vi "Team195_SetVoltageMotorControlOpenCANTalonSRX.vi"(4 "CAN.Max Vout":dbl=12.0, 5 "InverseTransformVIRef":T2, 6 "Invert":bool, 7 "TransformVIRef":T2, 8 "error in (no error)":errorcluster, 9 "Master Device Number":u8, 10 "Device Number":u8, 11 "Control Mode":T1) -> (0 "error out":errorcluster, 3 "MotorControlDeviceRef":T3={"DeviceStatus"={"status"=FALSE, "code"=0, "source"=""}, "Type"=enum."PWM", "PWM"={"Controller"=enum."Controller 1", "PWM Channel"=enum."Invalid", "DeadBand"={"Name"="", "maxPositivePwm"=0, "minPositivePwm"=0, "centerPwm"=0, "maxNegativePwm"=0, "minNegativePwm"=0, "angularRange"=0}}, "CAN"={"Device Number"=0, "Control Mode"=enum."Percent VBus", "Semaphore"=refnum, "Max Vout"=12.0, "TalonSRX Control Mode"=enum."Percent VBus"}, "Invert"=FALSE, "TransformRef"=refnum, "InvTransformRef"=refnum})   [LabVIEW 2014]
doc: "Creates a reference to the Victor motor controller you specify. You must open a reference before using any other VIs on this palette. After you open a reference to the Victor motor controller, you can use the SetOutput and GetOutput VIs to set and get the output voltage of the motor controller, respectively.\n\nThis software is licensed. Open the labview\\readme\\WPI Robotics Library Open Source License.txt file for more information."
uses:
  <vilib>/Rock Robotics/WPI/MotorControl/WPI_MotorControlDeviceRef.ctl
  <vilib>/Rock Robotics/WPI/MotorControl/WPI_MotorControlType.ctl
  <vilib>/Rock Robotics/SystemInterfaces/Typedef/FPGA_TypedefDigitalModule.ctl
  <vilib>/Rock Robotics/SystemInterfaces/DIO/FPGA_DIOPWMChannel.ctl
  <vilib>/Rock Robotics/WPI/PWM/WPI_PWMDeadband.ctl
  <vilib>/Rock Robotics/WPI/CAN/Jaguar/SubVIs/WPI_CANJaguar_ControlMode.ctl
  <vilib>/Rock Robotics/WPI/CAN/TalonSRX/WPI_CANTalonSRX_APIControlMode.ctl
  <vilib>/Rock Robotics/WPI/PWM/WPI_PWMTransform_ConPane.ctl
  <vilib>/Rock Robotics/SystemInterfaces/NetworkCommunication/NetComm_UsageReport_ResourceType.ctl
  <vilib>/Rock Robotics/WPI/CAN/TalonSRX/WPI_CANTalonSRX_GlobalOps.ctl
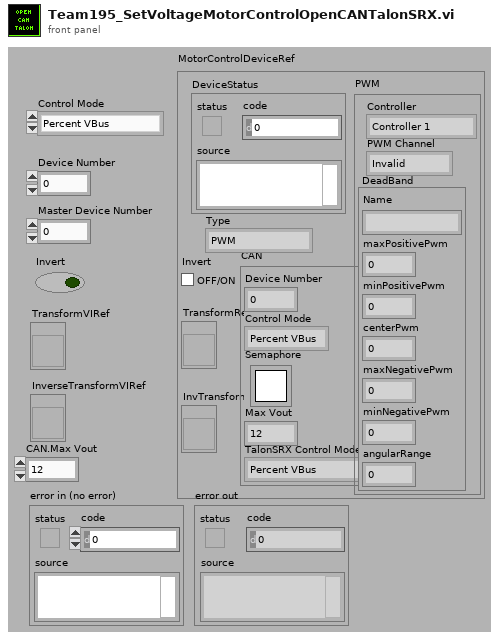
[diagram p1: front panel]
types:
  T1 = typedef "WPI_CANTalonSRX_APIControlMode.ctl" = enum8{"Percent VBus", "Speed", "Position", "Slave", "Unchanged / Invalid"}
  T2 = typedef "WPI_PWMTransform_ConPane.ctl" = refnum<vi>
  T3 = typedef "WPI_MotorControlDeviceRef.ctl" = cluster{"DeviceStatus":errorcluster, "Type":T4, "PWM":cluster{"Controller":T5, "PWM Channel":T6, "DeadBand":T7}, "CAN":cluster{"Device Number":u8, "Control Mode":T8, "Semaphore":T9, "Max Vout":dbl, "TalonSRX Control Mode":T1}, "Invert":bool, "TransformRef":T2, "InvTransformRef":T2}
  T4 = typedef "WPI_MotorControlType.ctl" = enum16{"PWM", "CAN", "CANTalonSRX"}
  T5 = typedef "FPGA_TypedefDigitalModule.ctl" = enum16{"Controller 1"}
  T6 = typedef "FPGA_DIOPWMChannel.ctl" = enum8{"PWM 0", "PWM 1", "PWM 2", "PWM 3", "PWM 4", "PWM 5", "PWM 6", "PWM 7", "PWM 8", "PWM 9", "PWM MXP 0", "PWM MXP 1", "PWM MXP 2", "PWM MXP 3", "PWM MXP 4", "PWM MXP 5", "PWM MXP 6", "PWM MXP 7", "PWM MXP 8", "PWM MXP 9", "Invalid"}
  T7 = typedef "WPI_PWMDeadband.ctl" = cluster{"Name":string, "maxPositivePwm":i32, "minPositivePwm":i32, "centerPwm":i32, "maxNegativePwm":i32, "minNegativePwm":i32, "angularRange":u16}
  T8 = typedef "WPI_CANJaguar_ControlMode.ctl" = enum8{"Percent VBus", "Current", "Speed", "Position", "Voltage"}
  T9 = typedef "Semaphore RefNum" = refnum<k1>
  T10 = typedef "WPI_CANTalonSRX_GlobalOps.ctl" = enum16{"Read For Send", "Write After Receive General", "Write After Receive Feedback", "Write After Receive Encoder", "Write After Receive Ain", "Write Error", "Get All", "Set Output", "Set Mode", "Set Master ID", "Set Brake Mode", "Set Reverse Feedback Sensor", "Set Reverse Closed Loop Output", "Set Override Limits", "Set Forward Limit Enabled", "Set Reverse Limit Enabled", "Set Feedback Select", "Set Profile Select", "Set Throttle Ramp Rate", "Disable"}
  T11 = typedef "NetComm_UsageReport_ResourceType.ctl" = enum8{"Controller", "Module", "Language", "CANPlugin", "Accelerometer", "ADXL345", "AnalogChannel", "AnalogTrigger", "AnalogTriggerOutput", "CANJaguar", "Compressor", "Counter", "Dashboard", "DigitalInput", "DigitalOutput", "DriverStationCIO", "DriverStationEIO", "DriverStationLCD", "Encoder", "GearTooth", "Gyro", "I2C", "Framework", "Jaguar", "Joystick", "Kinect", "KinectStick", "PIDController", "Preferences", "PWM", "Relay", "RobotDrive", "SerialPort", "Servo", "Solenoid", "SPI", "Task", "Ultrasonic", "Victor", "Button", "Command", "AxisCamera", "PCVideoServer", "SmartDashboard", "Talon", "HiTechnicColorSensor", "HiTechnicAccel", "HiTechnicCompass", "SRF08", "AnalogOutput", "Victor SP", "Talon SRX", "CAN Talon SRX"}
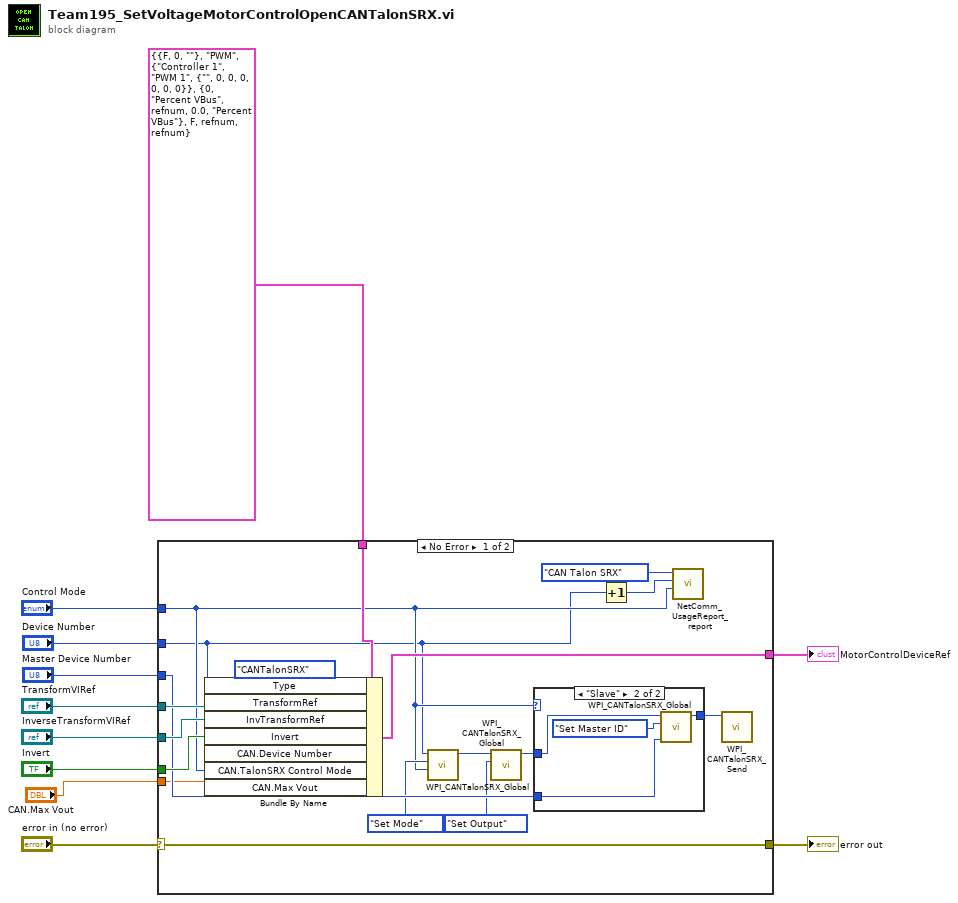
[diagram p0: block diagram]
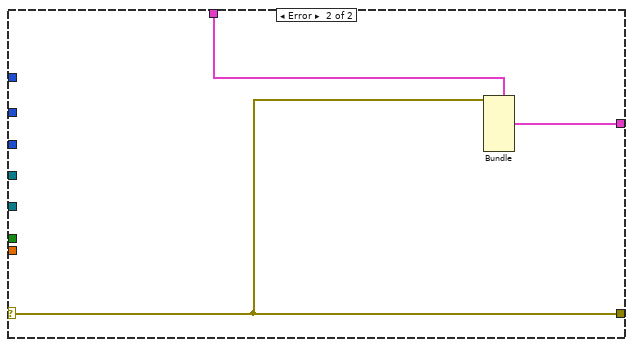
[diagram p3: hidden frame]
diagram:
  n1 = case shown="No Error" "error in (no error)" {
    selector: "error in (no error)" -> [w21 w35]
    tunnel: T3 {"DeviceStatus"={"status"=FALSE, "code"=0, "source"=""}, "Type"=enum."PWM", "PWM"={"Controller"=enum."Controller 1", "PWM Channel"=enum."PWM 1", "DeadBand"={"Name"="", "maxPositivePwm"=0, "minPositivePwm"=0, "centerPwm"=0, "maxNegativePwm"=0, "minNegativePwm"=0, "angularRange"=0}}, "CAN"={"Device Number"=0, "Control Mode"=enum."Percent VBus", "Semaphore"=refnum, "Max Vout"=0.0, "TalonSRX Control Mode"=enum."Percent VBus"}, "Invert"=FALSE, "TransformRef"=refnum, "InvTransformRef"=refnum} ("CAN Jaguar Ref Out") -> [w26 w37]
    tunnel: "InverseTransformVIRef" -> [w25 _]
    tunnel: "TransformVIRef" -> [w24 _]
    tunnel: "Invert" -> [w23 _]
    tunnel: "Device Number" -> [w17 _]
    tunnel: "Control Mode" -> [w18 _]
    tunnel: [w22 w36] -> w5
    tunnel: [w21 w35] -> w3
    tunnel: "Master Device Number" -> [w20 _]
    tunnel: "CAN.Max Vout" -> [w12 _]
    frame No Error {
      n2 = Bundle By Name(cluster=w26, "Type"=WPI_MotorControlType."CANTalonSRX", "TransformRef"=w24, "InvTransformRef"=w25, "Invert"=w23, "CAN.Device Number"=w17, "CAN.TalonSRX Control Mode"=w18, "CAN.Max Vout"=w12) -> (w22:T3)
      n3 = call <vilib>:"WPI_CANTalonSRX_Global.vi"("Control Mode"=w18, "Operation"=WPI_CANTalonSRX_GlobalOps."Set Mode", "Device ID (0)"=w17) -> ("Device ID Out"=w14:u8)  [unwired: 6 in, 2 out]
      n4 = call <vilib>:"WPI_CANTalonSRX_Global.vi"("Operation"=WPI_CANTalonSRX_GlobalOps."Set Output", "Device ID (0)"=w14) -> ("Device ID Out"=w13:u8)  [unwired: 7 in, 2 out]
      n5 = case shown="\"Slave\"" w18 {
        tunnel: w20 -> [_ w33]
        tunnel: w13 -> [w30 w32]
        tunnel: [w30 w31] -> w16
        frame Default {
        }
        frame "Slave" {
          n6 = call <vilib>:"WPI_CANTalonSRX_Global.vi"("Set Number"=w33, "Operation"=WPI_CANTalonSRX_GlobalOps."Set Master ID", "Device ID (0)"=w32) -> ("Device ID Out"=w31:u8)  [unwired: 6 in, 2 out]
        }
      }
      n7 = Increment(x=w17) -> (x+1=w28:u8)
      n8 = call <vilib>:"NetComm_UsageReport_report.vi"("Context"=w18, "Instance Number"=w28, "Resource Type"=NetComm_UsageReport_ResourceType."CAN Talon SRX") -> ()  [unwired: 9 in]
      n9 = call <vilib>:"WPI_CANTalonSRX_Send.vi"("Device ID (0)"=w16) -> ()  [unwired: 10 in, 1 out]
    }
    frame Error {
      n10 = Bundle(cluster=w37, "DeviceStatus"=w35) -> (w36:T3)  [unwired: 6 in]
    }
  }
  "MotorControlDeviceRef" <- w5
  "error out" <- w3
